vi "OSArchitecture.vi"(8 "error in (no error)":errorcluster) -> (0 "error out":errorcluster, 2 "32bit(T)/64bit(F)":bool)   [LabVIEW 2014]
panel:
  out "standard output":string
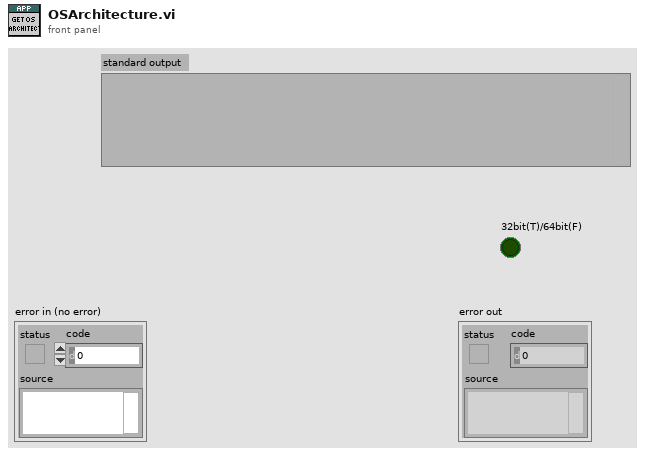
[diagram p1: front panel]
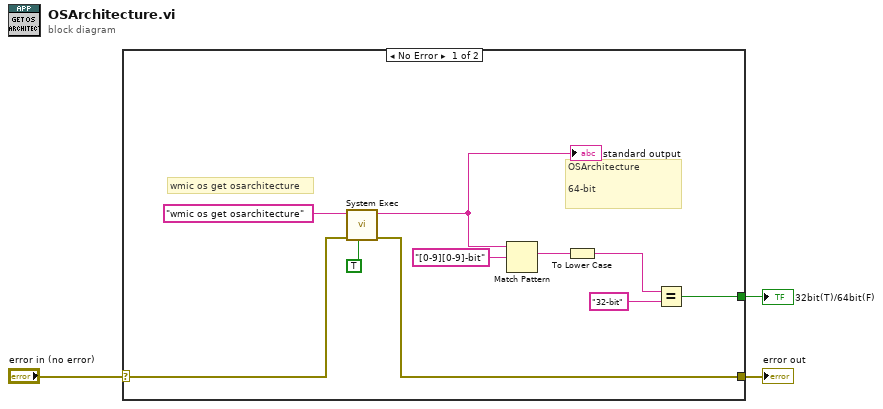
[diagram p0: block diagram]
diagram:
  n1 = case shown="No Error" "error in (no error)" {
    selector: "error in (no error)" -> [w10 w14]
    tunnel: [w9 w14] -> w2
    tunnel: [w6 _] -> w1
    frame No Error {
      # "OSArchitecture  \n\n64-bit"
      # "wmic os get osarchitecture"
      n2 = call <vilib>:"System Exec.vi"("run minimized? (F)"=TRUE, "error in (no error)"=w10, "command line"="wmic os get osarchitecture") -> ("error out"=w9:errorcluster, "standard output"=w12:string)  [unwired: 5 in, 2 out]
      "standard output" <- w12
      n3 = Match Pattern(string=w12, regular expression="[0-9][0-9]-bit") -> (match substring=w8:string)  [unwired: 1 in, 3 out]
      n4 = To Lower Case(string=w8) -> (all lower case string=w7:string)
      n5 = Equal?(x=w7, y="32-bit") -> (x = y?=w6:bool)
    }
    frame Error {
    }
  }
  "error out" <- w2
  "32bit(T)/64bit(F)" <- w1
